vi "set Defaults.vi"(0 "OBJ - Session in":refnum<class "Session - Root.lvclass">, 11 "error in":errorcluster) -> (4 "OBJ - Session out":refnum<class "Session - Root.lvclass">, 15 "error out":errorcluster)   [LabVIEW 2017, in "Session - Root.lvclass"]
doc: "OVERRIDE VI\nPlaceholder for decendant sessions to initialize and set their default values"
uses:
  Session - Root.lvclass
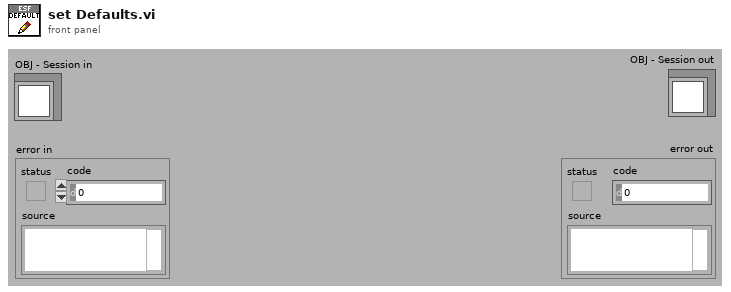
[diagram p1: front panel]
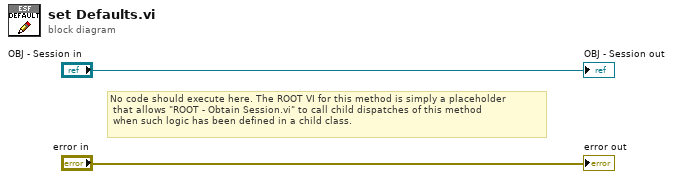
[diagram p0: block diagram]
diagram:
  # "No code should execute here. The ROOT VI for this method is simply a placeholder\n that allows \"ROOT - Obtain Session.vi\" to call child dispatches of this method\n when such logic has been defined in a child class."
  "error out" <- "error in"
  "OBJ - Session out" <- "OBJ - Session in"
